vi "New_VI.vi"(1 "Numeric":dbl) -> (0 "x+1":dbl)   [LabVIEW 2012]
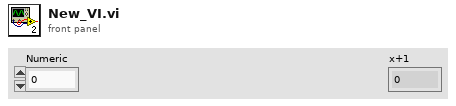
[diagram p1: front panel]
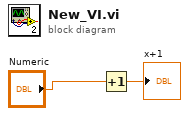
[diagram p0: block diagram]
diagram:
  n1 = Increment(x="Numeric") -> (x+1=→"x+1":dbl)
